vi "Datalog to ASCII (STATE).vi"(4 "Error in":errorcluster, 5 "ASCII output path":path=path "C:/Datalogs/Log1_S.txt", 6 "Precision":i16=4, 7 "Datalog path":path=path "C:/Datalogs/Log1_S.log") -> (0 "Error out":errorcluster)   [LabVIEW 2015]
uses:
  Ctls/All state values (for datalog).ctl
  Ctls/Environmental state values.ctl
  Ctls/Inertial state values.ctl
  <vilib>/Utility/file.llb/Write Delimited Spreadsheet (string).vi
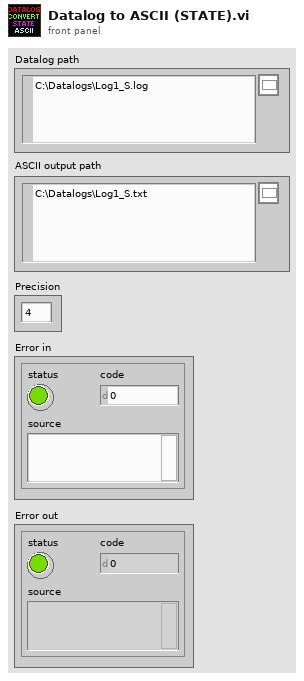
[diagram p1: front panel]
types:
  T1 = typedef "All state values (for datalog).ctl" = cluster{"Time Stamp":timestamp, "dt (ms)":i32, "Environmental state values":T2, "Inertial state values":T3}
  T2 = typedef "Environmental state values.ctl" = cluster{"Thermistor (degC)":sgl, "Sensor temp. (degC)":sgl, "P_atmos (Pa)":sgl, "Rel. Humidity (%)":sgl, "Density (kg/m^3)":sgl, "Dew point (degC)":sgl, "Pressure alt. (m)":sgl, "Density alt. (m)":sgl}
  T3 = typedef "Inertial state values.ctl" = cluster{"w_x (dps)":sgl, "w_y (dps)":sgl, "w_z (dps)":sgl, "a_x (g)":sgl, "a_y (g)":sgl, "a_z (g)":sgl, "Stale sample":u8, "Sensor temp. (degC)":sgl}
  T4 = enum16{"open", "replace", "create", "open or create", "replace or create", "replace or create with confirmation"}
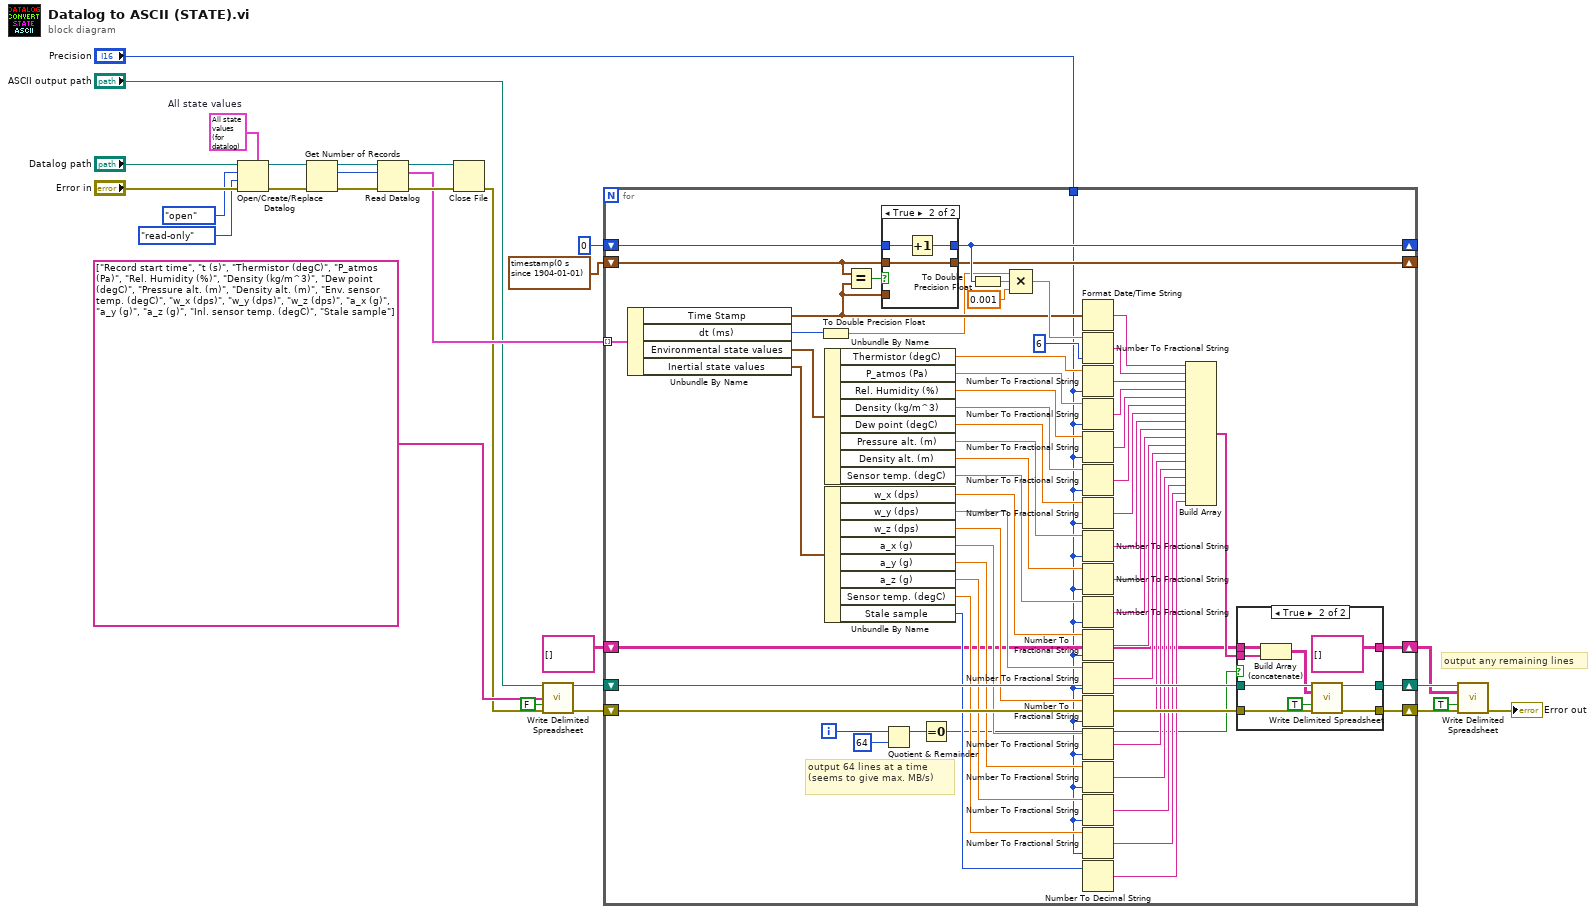
[diagram p0: block diagram]
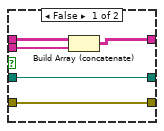
[diagram p2: hidden frame]
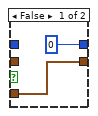
[diagram p3: hidden frame]
diagram:
  w13 = T1 {"Time Stamp"=timestamp(0 s since 1904-01-01), "dt (ms)"=0, "Environmental state values"={"Thermistor (degC)"=0.0, "Sensor temp. (degC)"=0.0, "P_atmos (Pa)"=0.0, "Rel. Humidity (%)"=0.0, "Density (kg/m^3)"=0.0, "Dew point (degC)"=0.0, "Pressure alt. (m)"=0.0, "Density alt. (m)"=0.0}, "Inertial state values"={"w_x (dps)"=0.0, "w_y (dps)"=0.0, "w_z (dps)"=0.0, "a_x (g)"=0.0, "a_y (g)"=0.0, "a_z (g)"=0.0, "Stale sample"=0, "Sensor temp. (degC)"=0.0}}  # All state values
  # "output any remaining lines"
  n1 = Open/Create/Replace Datalog(5:w13, 8:"Error in", 9:enum16{"read/write", "read-only", "write-only"}."read-only" ("access (0:read/write)"), 10:T4."open" ("operation (0:open)"), 11:"Datalog path") -> (0:w23:errorcluster, 3:w24:refnum<k1>)  [unwired: 1 in, 1 out]
  n2 = Get Number of Records(4:w23, 7:w24) -> (0:w20:errorcluster, 2:w21:i64, 3:w22:refnum<k1>)
  n3 = Read Datalog(4:w20, 6:w21, 7:w22) -> (0:w18:errorcluster, 2:w17:T1[], 3:w19:refnum<k1>)
  n4 = Close File(refnum=w19, error in=w18) -> (error out=w9:errorcluster)  [unwired: 1 out]
  n5 = call-poly <vilib>:"Write Delimited Spreadsheet.vi"("file path (dialog if empty)"="ASCII output path", "1D data"=string[] ["Record start time", "t (s)", "Thermistor (degC)", "P_atmos (Pa)", "Rel. Humidity (%)", "Density (kg/m^3)", "Dew point (degC)", "Pressure alt. (m)", "Density alt. (m)", "Env. sensor temp. (degC)", "w_x (dps)", "w_y (dps)", "w_z (dps)", "a_x (g)", "a_y (g)", "a_z (g)", "Inl. sensor temp. (degC)", "Stale sample"], "append to file? (F)"=FALSE, "error in (no error)"=w9) -> ("new file path (Not A Path if cancelled)"=w7:path, "error out"=w6:errorcluster)  [unwired: 10 in]
  n6 = for {
    tunnel: w17 -> [w63] mode=indexing
    tunnel: "Precision" -> [w29]
    shift-right: [w65] -> _
    shift-left: u32 0 -> [w66]
    shift-right: [w64] -> _
    shift-left: timestamp(0 s since 1904-01-01) ("Time stamp") -> [w67]
    shift-right: [w35] -> w5
    shift-left: w7 -> [w88]
    shift-right: [w34] -> w4
    shift-left: w6 -> [w89]
    shift-right: [w32] -> w1
    shift-left: string[][] [] -> [w31]
    i -> [w36]
    # "output 64 lines at a time (seems to give max. MB/s)"
    n7 = Unbundle By Name(w63) -> ("Time Stamp"=w62:timestamp, "dt (ms)"=w61:i32, "Environmental state values"=w59:T2, "Inertial state values"=w58:T3)
    n8 = To Double Precision Float(number=w61) -> (double precision float=w60:dbl)
    n9 = Unbundle By Name(w59) -> ("Thermistor (degC)"=w57:sgl, "P_atmos (Pa)"=w56:sgl, "Rel. Humidity (%)"=w55:sgl, "Density (kg/m^3)"=w54:sgl, "Dew point (degC)"=w53:sgl, "Pressure alt. (m)"=w52:sgl, "Density alt. (m)"=w51:sgl, "Sensor temp. (degC)"=w50:sgl)
    n10 = Unbundle By Name(w58) -> ("w_x (dps)"=w49:sgl, "w_y (dps)"=w48:sgl, "w_z (dps)"=w47:sgl, "a_x (g)"=w46:sgl, "a_y (g)"=w45:sgl, "a_z (g)"=w44:sgl, "Sensor temp. (degC)"=w43:sgl, "Stale sample"=w42:u8)
    n11 = Equal?(x=w67, y=w62) -> (x = y?=w68:bool)
    n12 = case shown="True" w68 {
      tunnel: [u32 0 w107] -> w65
      tunnel: w66 -> [_ w106]
      tunnel: w62 -> [w105 _]
      tunnel: w67 -> [_ w108]
      tunnel: [w105 w108] -> w64
      frame False {
      }
      frame True {
        n13 = Increment(x=w106) -> (x+1=w107:u32)
      }
    }
    n14 = Quotient & Remainder(x=w36, y=64) -> (x-y*floor(x/y)=w38:i32)  [unwired: 1 out]
    n15 = Equal To 0?(x=w38) -> (x = 0?=w30:bool)
    n16 = To Double Precision Float(number=w65) -> (double precision float=w87:dbl)
    n17 = Compound Arithmetic op=MULTIPLY(w60, w87, 0.001 ("value")) -> (w78:dbl)
    n18 = Format Date/Time String(seconds (now)=w62) -> (date/time string=w79:string)  [unwired: 2 in]
    n19 = Number To Fractional String(number=w78, precision (6)=i16 6) -> (F-format string=w77:string)  [unwired: 2 in]
    n20 = Number To Fractional String(number=w57, precision (6)=w29) -> (F-format string=w86:string)  [unwired: 2 in]
    n21 = Number To Fractional String(number=w56, precision (6)=w29) -> (F-format string=w85:string)  [unwired: 2 in]
    n22 = Number To Fractional String(number=w55, precision (6)=w29) -> (F-format string=w84:string)  [unwired: 2 in]
    n23 = Number To Fractional String(number=w54, precision (6)=w29) -> (F-format string=w83:string)  [unwired: 2 in]
    n24 = Number To Fractional String(number=w53, precision (6)=w29) -> (F-format string=w82:string)  [unwired: 2 in]
    n25 = Number To Fractional String(number=w52, precision (6)=w29) -> (F-format string=w81:string)  [unwired: 2 in]
    n26 = Number To Fractional String(number=w51, precision (6)=w29) -> (F-format string=w80:string)  [unwired: 2 in]
    n27 = Number To Fractional String(number=w50, precision (6)=w29) -> (F-format string=w76:string)  [unwired: 2 in]
    n28 = Number To Fractional String(number=w49, precision (6)=w29) -> (F-format string=w75:string)  [unwired: 2 in]
    n29 = Number To Fractional String(number=w48, precision (6)=w29) -> (F-format string=w74:string)  [unwired: 2 in]
    n30 = Number To Fractional String(number=w47, precision (6)=w29) -> (F-format string=w73:string)  [unwired: 2 in]
    n31 = Number To Fractional String(number=w46, precision (6)=w29) -> (F-format string=w72:string)  [unwired: 2 in]
    n32 = Number To Fractional String(number=w45, precision (6)=w29) -> (F-format string=w70:string)  [unwired: 2 in]
    n33 = Number To Fractional String(number=w44, precision (6)=w29) -> (F-format string=w69:string)  [unwired: 2 in]
    n34 = Number To Fractional String(number=w43, precision (6)=w29) -> (F-format string=w41:string)  [unwired: 2 in]
    n35 = Number To Decimal String(number=w42) -> (decimal integer string=w40:string)  [unwired: 1 in]
    n36 = Build Array(w79, w77, w86, w85, w84, w83, w82, w81, w80, w76, w75, w74, w73, w72, w70, w69, w41, w40) -> (w33:string[])
    n37 = case shown="True" w30 {
      tunnel: [w92 string[][] []] -> w32
      tunnel: [w91 w102] -> w35
      tunnel: [w90 w101] -> w34
      tunnel: w88 -> [w91 w99]
      tunnel: w89 -> [w90 w98]
      tunnel: w33 -> [w93 w97]
      tunnel: w31 -> [w94 w96]
      frame False {
        n38 = Build Array (concatenate)(w94, w93) -> (w92:string[][])
      }
      frame True {
        n39 = Build Array (concatenate)(w96, w97) -> (w95:string[][])
        n40 = call-poly <vilib>:"Write Delimited Spreadsheet.vi"("file path (dialog if empty)"=w99, "2D data"=w95, "append to file? (F)"=TRUE, "error in (no error)"=w98) -> ("new file path (Not A Path if cancelled)"=w102:path, "error out"=w101:errorcluster)  [unwired: 10 in]
      }
    }
  }
  n41 = call-poly <vilib>:"Write Delimited Spreadsheet.vi"("file path (dialog if empty)"=w5, "2D data"=w1, "append to file? (F)"=TRUE, "error in (no error)"=w4) -> ("error out"=→"Error out":errorcluster)  [unwired: 10 in, 1 out]
